vi "Find VidRec folder.vi"(8 "error in (no error)":errorcluster, 11 "Timelapse folder path":path) -> (0 "error out":errorcluster, 3 "appended path":path)   [LabVIEW 2020]
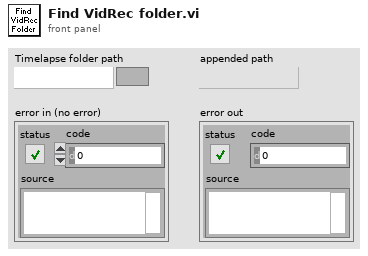
[diagram p1: front panel]
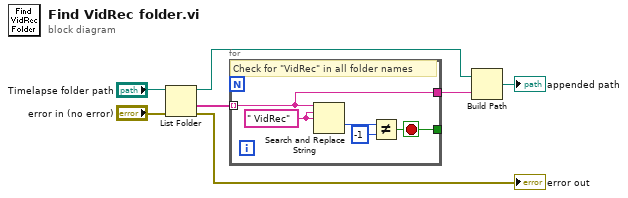
[diagram p0: block diagram]
diagram:
  n1 = List Folder(path="Timelapse folder path", error in="error in (no error)") -> (path out=w3:path, folder names=w2:string[], error out=→"error out":errorcluster)  [unwired: 2 in, 1 out]
  n2 = for {
    tunnel: w2 -> [w8] mode=indexing
    tunnel: [w9] -> _
    tunnel: [w8] -> w4
    stop <- w9 stop-if-true
    w12 = " VidRec" ("string")
    # "Check for \"VidRec\" in all folder names"
    n3 = Search and Replace String(input string=w8, search string=w12, replace string=w12) -> (offset past replacement=w11:i32)  [unwired: 5 in, 3 out]
    n4 = Not Equal?(x=w11, y=-1) -> (x != y?=w9:bool)
  }
  n5 = Build Path(base path=w3, name or relative path=w4) -> (appended path=→"appended path":path)
